vi "Top-V2.2.vi"() -> ()   [LabVIEW 2014]
uses:
  BackMapGlobalV2.2.vi
  ShowMapGlobalV2.2.vi
panel:
  out "Buttom List":string[][](array[string])=[["", "P1", "P2"], ["↑", "\u0000", ""], ["←", "\u0000", ""], ["↓", "", ""], ["→", "", ""], ["☆", "", ""], ["★", "", ""]]
  out "ButtonStringArray":string[](array[string])
  in  "SkipButtonReset?":bool
  out "ButtonArray":i32[](array[numeric])
  out "ButtonSetDone?":bool
  in  "Start":bool
  out "NotFirstClick?":bool
  out "FirstClikPosition":i32[](array[numeric])
  out "Message":string="Please set length, width, number of mines. And press\"SET UP\"."
  in  "Set OK":bool
  out "P2's Score":i32
  out "P1's Score":i32
  out "Mines Remain":i32
  in  "Number of Total Mines":i32(knob)=99 scale=1.0..100.0
  out "SamePlace?":bool
  out "ZeroListBefore":i32[][](array[numeric])
  out "WhichPlayer":i32
  out "ZeroList":i32[][](array[numeric])
  out "BackMap":i32[][](array[numeric])
  in  "Number of Columns":i32(slide)=30 scale=0.0..30.0
  in  "Number of Rows":i32(slide)=16 scale=0.0..16.0
  out "Position":i32[][](array[numeric])=[[0, 1], [1, 0]]
  out "Show Map":cluster{"Color Box":u32, "String":string}[][](array[cluster])=[[{"Color Box"=6908265, "String"=""}]]
  in  "Leave":bool
  out "Char":i16
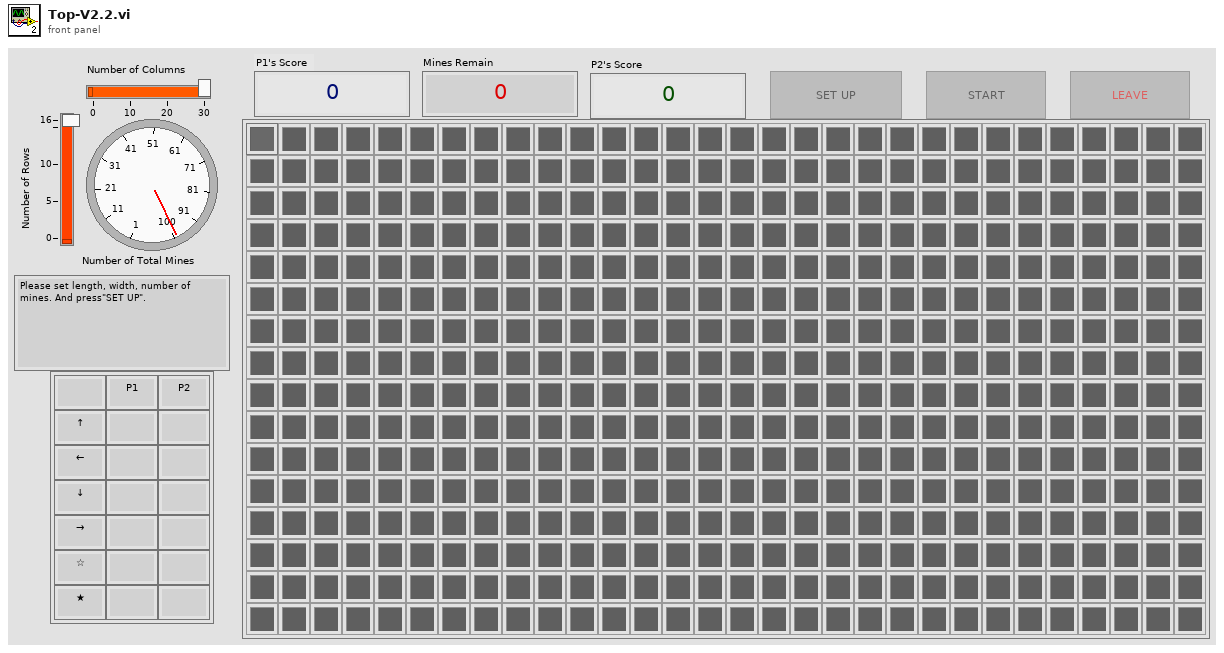
[diagram p1: front panel]
types:
  T1 = enum16{"int", "wait buttom", "w", "a", "s", "d", "q", "e", "i", "j", "k", "l", "u", "o", "spare", "ZeroSpread"}
  T2 = enum8{"Enabled", "Disabled", "Disabled and Grayed Out"}
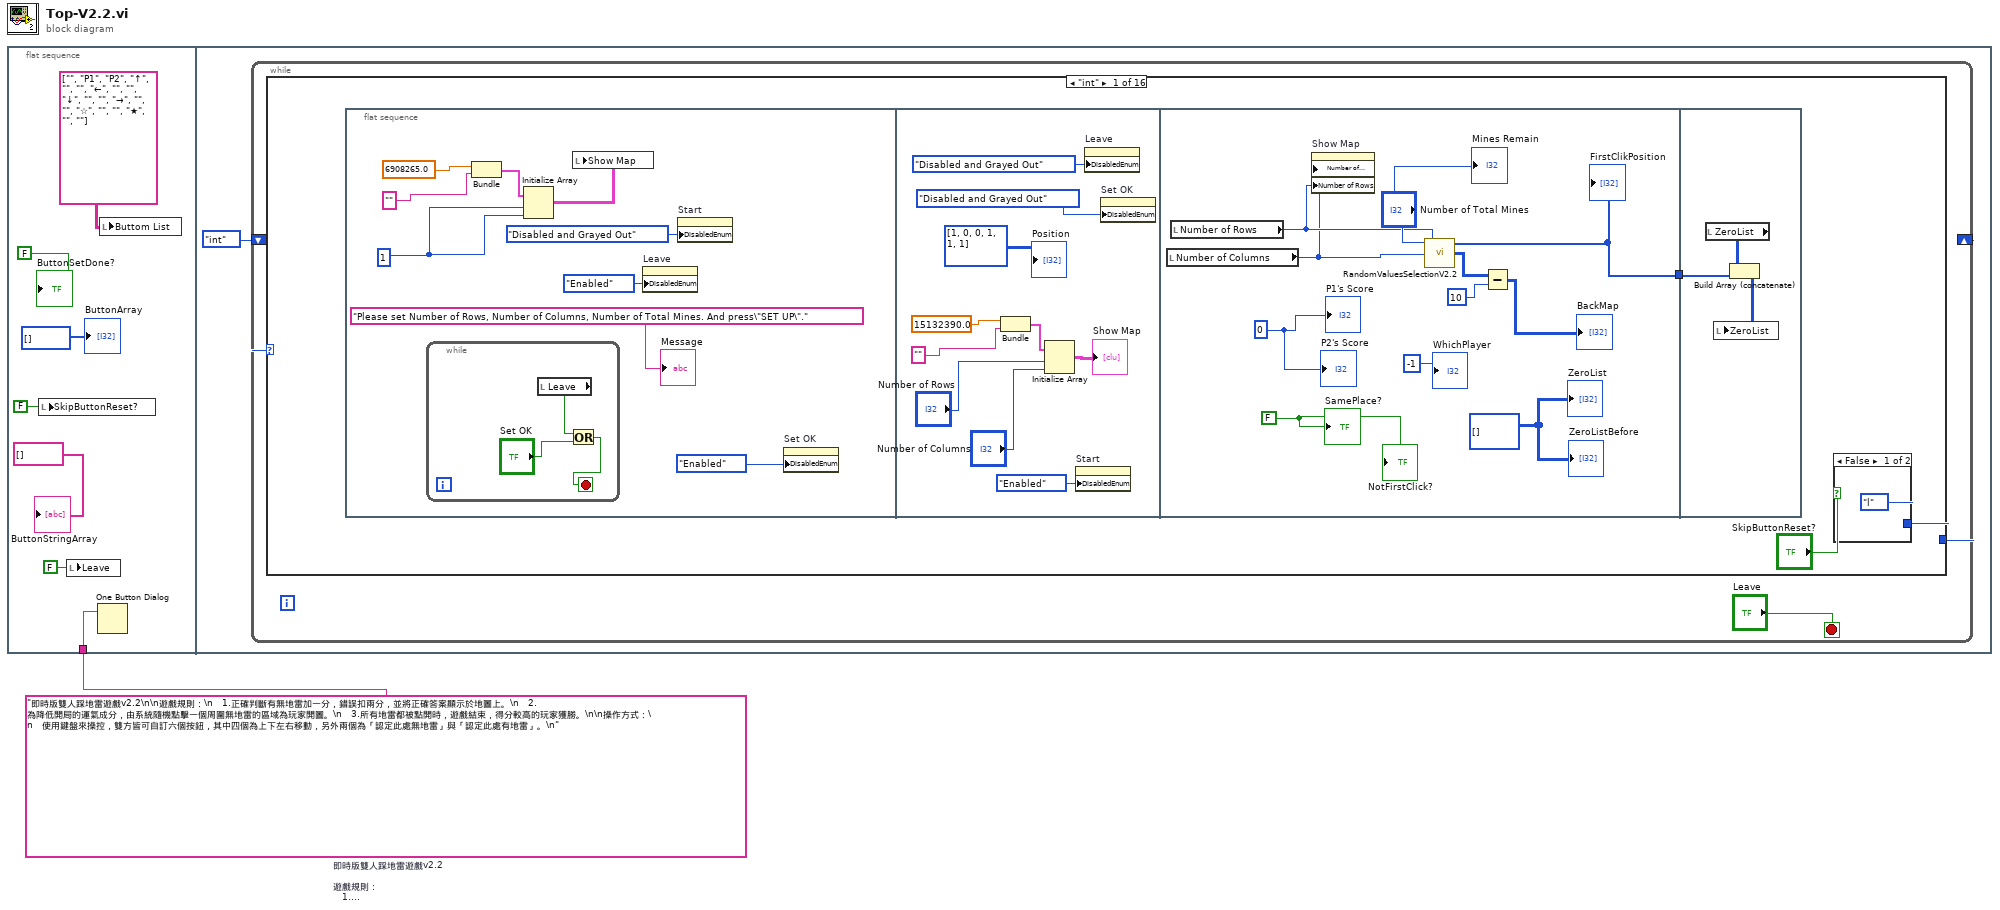
[diagram p0: block diagram]
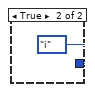
[diagram p2: hidden frame]
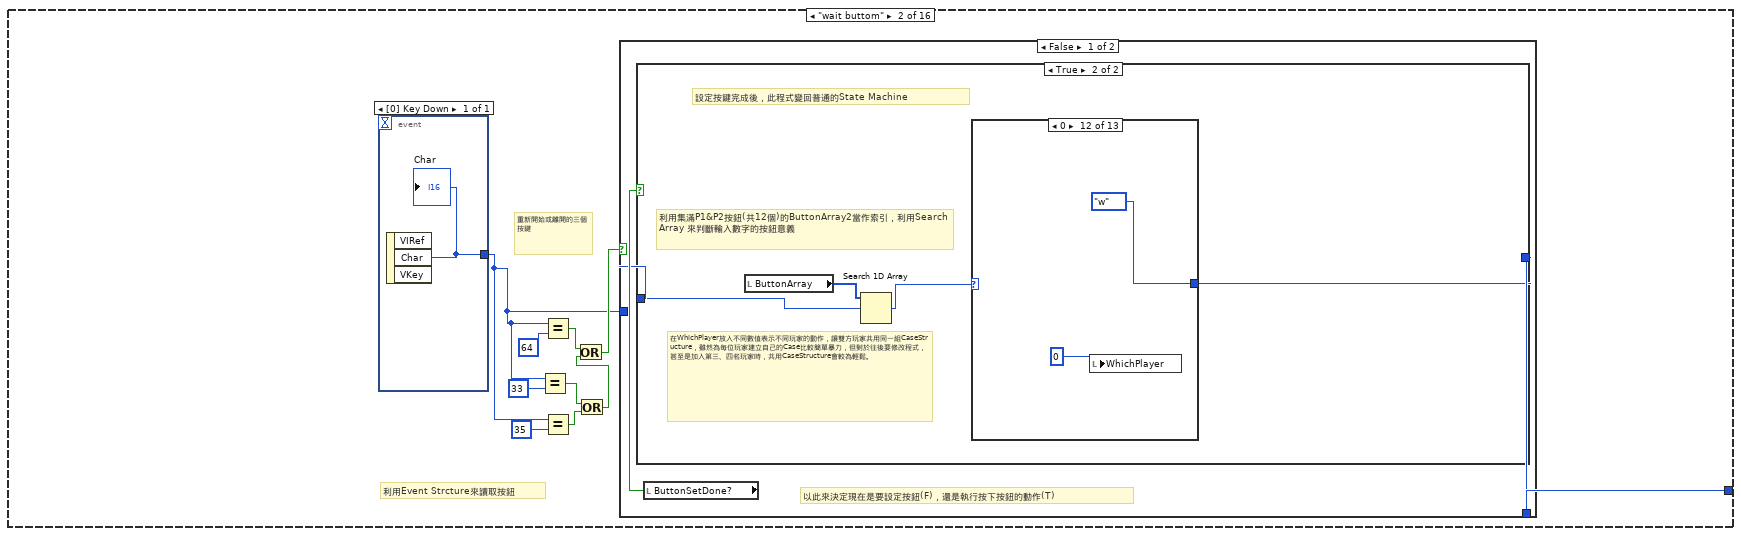
[diagram p3: hidden frame]
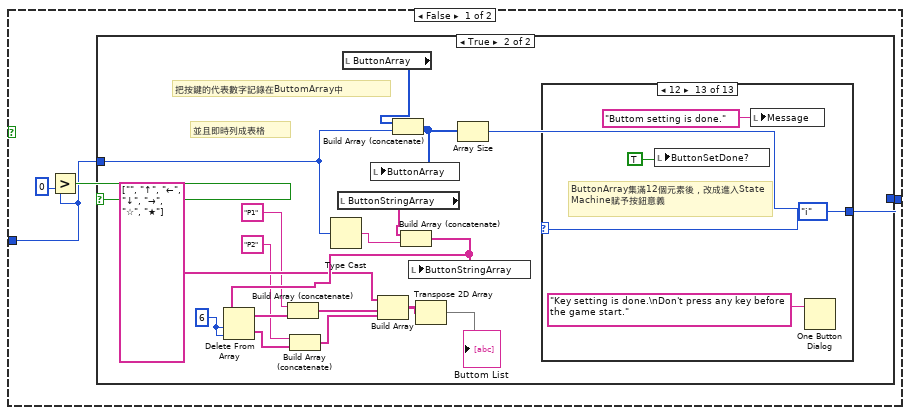
[diagram p4: hidden frame]
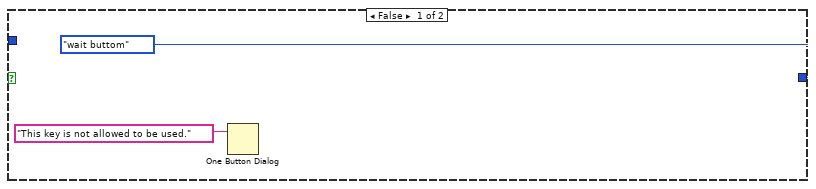
[diagram p5: hidden frame]
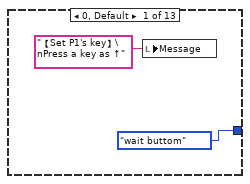
[diagram p6: hidden frame]
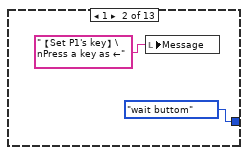
[diagram p7: hidden frame]
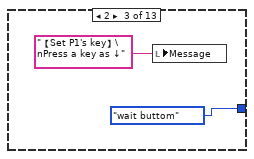
[diagram p8: hidden frame]
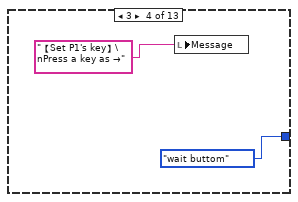
[diagram p9: hidden frame]
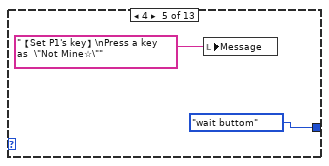
[diagram p10: hidden frame]
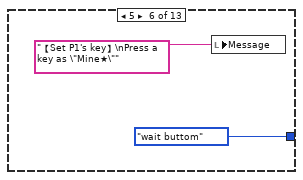
[diagram p11: hidden frame]
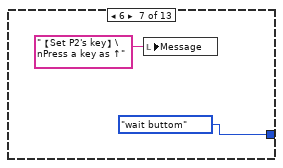
[diagram p12: hidden frame]
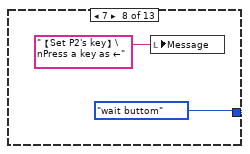
[diagram p13: hidden frame]
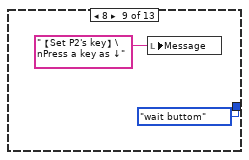
[diagram p14: hidden frame]
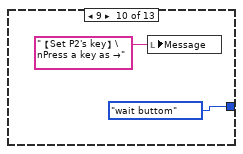
[diagram p15: hidden frame]
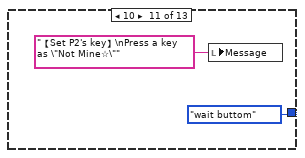
[diagram p16: hidden frame]
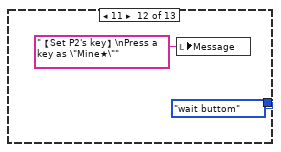
[diagram p17: hidden frame]
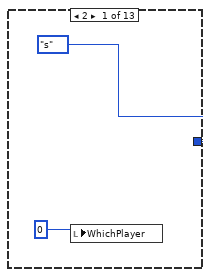
[diagram p18: hidden frame]
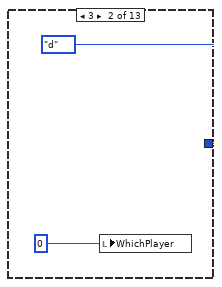
[diagram p19: hidden frame]
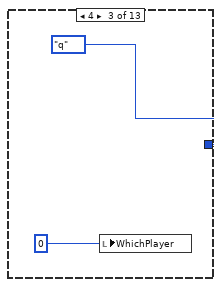
[diagram p20: hidden frame]
diagram:
  w1 = "即時版雙人踩地雷遊戲v2.2\n\n遊戲規則：\n　1.正確判斷有無地雷加一分，錯誤扣兩分，並將正確答案顯示於地圖上。\n　2.為降低開局的運氣成分，由系統隨機點擊一個周圍無地雷的區域為玩家開圖。\n　3.所有地雷都被點開時，遊戲結束，得分較高的玩家獲勝。\n\n操作方式：\n　使用鍵盤來操控，雙方皆可自訂六個按鈕，其中四個為上下左右移動，另外兩個為「認定此處無地雷」與「認定此處有地雷」。\n"  # 即時版雙人踩地雷遊戲v2.2  遊戲規則： 　1.正確判斷有無地雷加一分，錯誤扣兩分，並將正確答案顯示於地圖上。 　2.為降低開局的運氣成分，由系統隨機點擊一個周圍無地雷的區域為玩家開圖。 　3.所有地雷都被點開時，遊戲結束，得分較高的玩家獲勝。  操作方式： 　使用鍵盤來操控，雙方皆可自訂六個按鈕，其中四個為上下左右移動，另外兩個為「認定此處無地雷」與「認定此處有地雷」。
  n1 = flat-sequence {
    tunnel: w1 -> [w4]
    frame #0 {
      n2 = local write "SkipButtonReset?"(FALSE ("SkipButtomReset?")) -> ()
      n3 = local write "Leave"(FALSE ("Leave")) -> ()
      n4 = One Button Dialog(message=w4) -> ()  [unwired: 1 in, 1 out]
      n5 = local write "Buttom List"(string[][] [["", "P1", "P2"], ["↑", "", ""], ["←", "", ""], ["↓", "", ""], ["→", "", ""], ["☆", "", ""], ["★", "", ""]]) -> ()
      "ButtonSetDone?" <- FALSE ("SetButtom?")
      "ButtonArray" <- i32[] []
      "ButtonStringArray" <- string[] []
    }
    frame #1 {
      n6 = while {
        shift-right: [w10] -> _
        shift-left: T1."int" -> [w11]
        stop <- "Leave" stop-if-true
        n7 = case shown="\"int\"" w11 {
          tunnel: [w15 w63 T1."wait buttom" T1."wait buttom" T1."wait buttom" T1."wait buttom" w356 w465 w597 T1."wait buttom" T1."wait buttom" T1."wait buttom" T1."wait buttom" T1."wait buttom" T1."wait buttom" w645] -> w10
          frame "int" {
            n8 = flat-sequence {
              tunnel: [w42] -> w14
              tunnel: w14 -> [w52]
              frame #0 {
                w21 = 1 ("dimension size")
                n9 = while {
                  stop <- w27 stop-if-true
                  n10 = local read "Leave"() -> (w29:bool)
                  n11 = Or(x=w29, y="Set OK") -> (x .or. y?=w27:bool)
                }
                n12 = Bundle(6908265.0, "") -> (w24:cluster{dbl, string})  [unwired: 1 in]
                n13 = Initialize Array(w24, w21, w21) -> (w22:cluster{dbl, string}[][])
                n14 = local write "Show Map"(w22) -> ()
                n15 = property on="Leave" class="Bool (strict)"("DisabledEnum"=T2."Enabled" ("Disabled")) -> ()  [unwired: 2 in, 2 out]
                n16 = property on="Start" class="Bool (strict)"("DisabledEnum"=T2."Disabled and Grayed Out" ("Disabled")) -> ()  [unwired: 2 in, 2 out]
                n17 = property on="Set OK" class="Bool (strict)"("DisabledEnum"=T2."Enabled" ("Disabled")) -> ()  [unwired: 2 in, 2 out]
                "Message" <- "Please set Number of Rows, Number of Columns, Number of Total Mines. And press\"SET UP\"."
              }
              frame #1 {
                n18 = Bundle(15132390.0, "") -> (w37:cluster{dbl, string})  [unwired: 1 in]
                n19 = Initialize Array(w37, "Number of Rows", "Number of Columns") -> (→"Show Map":cluster{dbl, string}[][])
                n20 = property on="Start" class="Bool (strict)"("DisabledEnum"=T2."Enabled" ("Disabled")) -> ()  [unwired: 2 in, 2 out]
                n21 = property on="Leave" class="Bool (strict)"("DisabledEnum"=T2."Disabled and Grayed Out" ("Disabled")) -> ()  [unwired: 2 in, 2 out]
                n22 = property on="Set OK" class="Bool (strict)"("DisabledEnum"=T2."Disabled and Grayed Out" ("Disabled")) -> ()  [unwired: 2 in, 2 out]
                "Position" <- i32[][] [[1, 0], [0, 1], [1, 1]]
              }
              frame #2 {
                w43 = FALSE
                w44 = i32[][] []
                w46 = 0 ("P1's Score")
                n23 = local read "Number of Columns"() -> (w40:i32)
                n24 = local read "Number of Rows"() -> (w41:i32)
                n25 = property on="Show Map" class="Arr (strict)"("Number of Columns"=w40, "Number of Rows"=w41) -> ()  [unwired: 2 in, 2 out]
                n26 = call "RandomValuesSelectionV2.2.vi"("Number of Columns"=w40, "Number of  Rows"=w41, "Number of Mine"="Number of Total Mines") -> ("FullMap"=w48:i32[][], "FirstClikPosition"=w42:i32[])  [unwired: 2 in]
                "FirstClikPosition" <- w42
                n27 = Subtract(x=w48, y=10) -> (x-y=→"BackMap":i32[][])
                "Mines Remain" <- "Number of Total Mines"
                "P1's Score" <- w46
                "P2's Score" <- w46
                "ZeroList" <- w44
                "WhichPlayer" <- -1
                "ZeroListBefore" <- w44
                "SamePlace?" <- w43
                "NotFirstClick?" <- w43
              }
              frame #3 {
                n28 = local read "ZeroList"() -> (w53:i32[][])
                n29 = Build Array (concatenate)(w53, w52) -> (w51:i32[][])
                n30 = local write "ZeroList"(w51) -> ()
              }
            }
            n31 = case shown="False" "SkipButtonReset?" {
              tunnel: [T1."l" T1."i"] -> w15
              frame False {
              }
              frame True {
              }
            }
          }
          frame "wait buttom" {
            # "重新開始或離開的三個按鍵"
            # "利用Event Strcture來讀取按鈕"
            n32 = event shown="[0] Key Down" {
              selector: _ -> [_]
              dyn-events: _ -> [_]
              timeout: _ -> [_]
              tunnel: [w157] -> w58
              event Key Down {
                n33 = event-data() -> ("Char"=w157:i16)  [unwired: 1 in, 2 out]
                "Char" <- w157
              }
            }
            n34 = Equal?(x=w58, y=i16 33) -> (x = y?=w55:bool)
            n35 = Equal?(x=w58, y=i16 64) -> (x = y?=w60:bool)
            n36 = Equal?(x=w58, y=i16 35) -> (x = y?=w56:bool)
            n37 = Or(x=w55, y=w56) -> (x .or. y?=w54:bool)
            n38 = Or(x=w60, y=w54) -> (x .or. y?=w59:bool)
            n39 = case shown="False" w59 {
              tunnel: [w64 w148] -> w63
              tunnel: w58 -> [w65 w149]
              frame False {
                # "以此來決定現在是要設定按鈕(F)，還是執行按下按鈕的動作(T)"
                n40 = local read "ButtonSetDone?"() -> (w66:bool)
                n41 = case shown="True" w66 {
                  tunnel: w65 -> [w68 w120]
                  tunnel: [w67 w122] -> w64
                  frame False {
                    n42 = Greater?(x=w68, y=i16 0) -> (0:w69:bool)
                    n43 = case shown="True" w69 {
                      tunnel: w68 -> [_ w86]
                      tunnel: [T1."wait buttom" w88] -> w67
                      frame False {
                        n44 = One Button Dialog(message="This key is not allowed to be used.") -> ()  [unwired: 1 in, 1 out]
                      }
                      frame True {
                        w82 = 6 ("index")
                        # "並且即時列成表格"
                        # "把按鍵的代表數字記錄在ButtomArray中"
                        n45 = Type Cast(x=w86) -> (*(type *) &x=w84:string)  [unwired: 1 in]
                        n46 = local read "ButtonStringArray"() -> (w85:string[])
                        n47 = local read "ButtonArray"() -> (w90:i32[])
                        n48 = Build Array (concatenate)(w90, w86) -> (w87:i32[])
                        n49 = local write "ButtonArray"(w87) -> ()
                        n50 = Build Array (concatenate)(w85, w84) -> (w83:string[])
                        n51 = Delete From Array(array=w83, length=w82, index=w82) -> (deleted portion=w74:string[], array with subset deleted=w77:string[])
                        n52 = Build Array (concatenate)("P1", w77) -> (w76:string[])
                        n53 = Build Array (concatenate)("P2", w74) -> (w73:string[])
                        n54 = Build Array(string[] ["", "↑", "←", "↓", "→", "☆", "★"], w76, w73) -> (w80:string[][])
                        n55 = local write "ButtonStringArray"(w83) -> ()
                        n56 = Transpose 2D Array(2D array=w80) -> (transposed array=→"Buttom List":string[][])
                        n57 = Array Size(array=w87) -> (size(s)=w89:i32)
                        n58 = case shown="12" w89 {
                          tunnel: [T1."wait buttom" T1."wait buttom" T1."wait buttom" T1."wait buttom" T1."wait buttom" T1."wait buttom" T1."wait buttom" T1."wait buttom" T1."wait buttom" T1."wait buttom" T1."wait buttom" T1."wait buttom" T1."i"] -> w88
                          frame 0, Default {
                            n59 = local write "Message"("【Set P1's key】\nPress a key as ↑" ("Message")) -> ()
                          }
                          frame 1 {
                            n60 = local write "Message"("【Set P1's key】\nPress a key as ←" ("Message")) -> ()
                          }
                          frame 2 {
                            n61 = local write "Message"("【Set P1's key】\nPress a key as ↓" ("Message")) -> ()
                          }
                          frame 3 {
                            n62 = local write "Message"("【Set P1's key】\nPress a key as →" ("Message")) -> ()
                          }
                          frame 4 {
                            n63 = local write "Message"("【Set P1's key】\nPress a key as  \"Not Mine☆\"" ("Message")) -> ()
                          }
                          frame 5 {
                            n64 = local write "Message"("【Set P1's key】\nPress a key as \"Mine★\"" ("Message")) -> ()
                          }
                          frame 6 {
                            n65 = local write "Message"("【Set P2's key】\nPress a key as ↑" ("Message")) -> ()
                          }
                          frame 7 {
                            n66 = local write "Message"("【Set P2's key】\nPress a key as ←" ("Message")) -> ()
                          }
                          frame 8 {
                            n67 = local write "Message"("【Set P2's key】\nPress a key as ↓" ("Message")) -> ()
                          }
                          frame 9 {
                            n68 = local write "Message"("【Set P2's key】\nPress a key as →" ("Message")) -> ()
                          }
                          frame 10 {
                            n69 = local write "Message"("【Set P2's key】\nPress a key as \"Not Mine☆\"" ("Message")) -> ()
                          }
                          frame 11 {
                            n70 = local write "Message"("【Set P2's key】\nPress a key as \"Mine★\"" ("Message")) -> ()
                          }
                          frame 12 {
                            # "ButtonArray集滿12個元素後，改成進入State Machine賦予按鈕意義"
                            n71 = local write "ButtonSetDone?"(TRUE ("SetButtom?")) -> ()
                            n72 = local write "Message"("Buttom setting is done." ("Message")) -> ()
                            n73 = One Button Dialog(message="Key setting is done.\nDon't press any key before the game start.") -> ()  [unwired: 1 in, 1 out]
                          }
                        }
                      }
                    }
                  }
                  frame True {
                    # "在WhichPlayer放入不同數值表示不同玩家的動作，讓雙方玩家共用同一組CaseStructure，雖然為每位玩家建立自己的Case比較簡單暴力，但對於往後要修改程式，甚至是加入第三、四名玩家時，共用CaseStructure會較為輕鬆。"
                    # "利用集滿P1&P2按鈕(共12個)的ButtonArray2當作索引，利用Search Array 來判斷輸入數字的按鈕意義"
                    # "設定按鍵完成後，此程式變回普通的State Machine"
                    n74 = local read "ButtonArray"() -> (w121:i32[])
                    n75 = Search 1D Array(1D array=w121, element=w120) -> (index of element=w119:i32)  [unwired: 1 in]
                    n76 = case shown="0" w119 {
                      tunnel: [T1."s" T1."d" T1."q" T1."e" T1."w" T1."a" T1."s" T1."d" T1."q" T1."e" T1."wait buttom" T1."w" T1."a"] -> w122
                      frame 2 {
                        n77 = local write "WhichPlayer"(0 ("WhichPlayer")) -> ()
                      }
                      frame 3 {
                        n78 = local write "WhichPlayer"(0 ("WhichPlayer")) -> ()
                      }
                      frame 4 {
                        n79 = local write "WhichPlayer"(0 ("WhichPlayer")) -> ()
                      }
                      frame 5 {
                        n80 = local write "WhichPlayer"(0 ("WhichPlayer")) -> ()
                      }
                      frame 6 {
                        n81 = local write "WhichPlayer"(1 ("WhichPlayer")) -> ()
                      }
                      frame 7 {
                        n82 = local write "WhichPlayer"(1 ("WhichPlayer")) -> ()
                      }
                      frame 8 {
                        n83 = local write "WhichPlayer"(1 ("WhichPlayer")) -> ()
                      }
                      frame 9 {
                        n84 = local write "WhichPlayer"(1 ("WhichPlayer")) -> ()
                      }
                      frame 10 {
                        n85 = local write "WhichPlayer"(1 ("WhichPlayer")) -> ()
                      }
                      frame 11 {
                        n86 = local write "WhichPlayer"(1 ("WhichPlayer")) -> ()
                      }
                      frame -1, Default {
                      }
                      frame 0 {
                        n87 = local write "WhichPlayer"(0 ("WhichPlayer")) -> ()
                      }
                      frame 1 {
                        n88 = local write "WhichPlayer"(0 ("WhichPlayer")) -> ()
                      }
                    }
                  }
                }
              }
              frame True {
                n89 = case shown="35" w149 {
                  tunnel: [T1."spare" T1."int" T1."wait buttom" T1."int"] -> w148
                  frame 64 {
                    n90 = local write "Leave"(TRUE ("Leave")) -> ()
                  }
                  frame 35 {
                    n91 = local write "SkipButtonReset?"(TRUE ("SkipButtomReset?")) -> ()
                  }
                  frame -1, Default {
                  }
                  frame 33 {
                    n92 = local write "SkipButtonReset?"(FALSE ("SkipButtomReset?")) -> ()
                  }
                }
              }
            }
          }
          frame "w" {
            n93 = flat-sequence {
              tunnel: [w170] -> w159
              tunnel: w159 -> [w193]
              tunnel: [w193] -> w158
              tunnel: w158 -> [w197]
              frame #0 {
                n94 = local read "WhichPlayer"() -> (w161:i32)
                n95 = local read "BackMap"() -> (w164:i32[][])
                n96 = local read "Position"() -> (w171:i32[][])
                n97 = local read "SamePlace?"() -> (w168:bool)
                n98 = Index Array(array=w171, index (row) #1=w161, index (col) #1=0 ("index (row)"), index (row) #2=w161, index (col) #2=1 ("disabled index (col)")) -> (element #1=w163:i32, element #2=w162:i32)
                n99 = call "AfterSamePositionColor-V2.2.vi"("WhichPlayer"=w161, "index (col)"=w162, "index (row)"=w163, "BackMap"=w164) -> ("Numeric"=w167:dbl)  [unwired: 2 in]
                n100 = call "ToBackMap-V2.2.vi"("Column"=w162, "Row"=w163, "BackMap"=w164) -> ("String"=w169:string, "Numeric"=w166:dbl)  [unwired: 2 in]
                n101 = Select(t=w167, s=w168, f=w166) -> (s? t:f=w165:dbl)
                n102 = Greater?(x=w163, y=0) -> (0:w174:bool)
                n103 = case shown="True" w174 {
                  tunnel: w163 -> [_ w191]
                  tunnel: w171 -> [w176 w182]
                  tunnel: [w176 w188] -> w170
                  tunnel: w165 -> [_ w179]
                  tunnel: w169 -> [_ w178]
                  tunnel: w161 -> [_ w177]
                  frame False {
                  }
                  frame True {
                    n104 = Decrement(x=w191) -> (x-1=w189:i32)
                    n105 = local read "Show Map"() -> (w181:cluster{"Color Box":u32, "String":string}[][])
                    n106 = Bundle("Numeric"=w179, "String"=w178) -> (w183:cluster{"Numeric":dbl, "String":string})  [unwired: 1 in]
                    n107 = Index Array(array=w182, index (row) #1=w177, index (col) #1=0 ("index (row)"), index (row) #2=w177, index (col) #2=1 ("disabled index (col)")) -> (element #1=w186:i32, element #2=w187:i32)
                    n108 = Replace Array Subset(array=w182, new element=w189, index (row)=w177, index (col)=0 ("index (row)")) -> (w188:i32[][])
                    n109 = Replace Array Subset(array=w181, new element=w183, index (row)=w186, index (col)=w187) -> (w180:cluster{"Color Box":u32, "String":string}[][])
                    n110 = local write "Show Map"(w180) -> ()
                  }
                }
              }
              frame #1 {
                n111 = local write "SamePlace?"(FALSE ("SamePlace?")) -> ()
              }
              frame #2 {
                n112 = local read "WhichPlayer"() -> (w198:i32)
                n113 = local write "Position"(w197) -> ()
                n114 = local read "BackMap"() -> (w202:i32[][])
                n115 = Index Array(array=w197, index (row) #1=w198, index (col) #1=0 ("index (row)"), index (row) #2=w198, index (col) #2=1 ("disabled index (col)")) -> (element #1=w201:i32, element #2=w200:i32)
                n116 = call "ZeroOrNot-V2.2.vi"("WhichPlayer"=w198, "index (col)"=w200, "index (row)"=w201, "BackMap"=w202) -> ("Numeric"=w196:dbl)  [unwired: 2 in]
                n117 = call "PositionSameOrNot-V2.2.vi"("BlueOrGreen"=w196, "Position"=w197) -> ("SamePosition?"=w194:bool, "FinalColor"=w195:dbl)  [unwired: 1 in]
                n118 = local read "Show Map"() -> (w206:cluster{"Color Box":u32, "String":string}[][])
                n119 = local write "SamePlace?"(w194) -> ()
                n120 = call "ToBackMap-V2.2.vi"("Column"=w200, "Row"=w201, "BackMap"=w202) -> ("String"=w203:string)  [unwired: 2 in, 1 out]
                n121 = Bundle("FinalColor"=w195, "String"=w203) -> (w205:cluster{"FinalColor":dbl, "String":string})  [unwired: 1 in]
                n122 = Replace Array Subset(array=w206, new element=w205, index (row)=w201, index (col)=w200) -> (w207:cluster{"Color Box":u32, "String":string}[][])
                n123 = local write "Show Map"(w207) -> ()
              }
            }
          }
          frame "a" {
            n124 = flat-sequence {
              tunnel: [w221] -> w209
              tunnel: w209 -> [w241]
              tunnel: [w241] -> w208
              tunnel: w208 -> [w245]
              frame #0 {
                n125 = local read "BackMap"() -> (w216:i32[][])
                n126 = local read "WhichPlayer"() -> (w213:i32)
                n127 = local read "SamePlace?"() -> (w218:bool)
                n128 = local read "Position"() -> (w222:i32[][])
                n129 = Index Array(array=w222, index (row) #1=w213, index (col) #1=0 ("index (row)"), index (row) #2=w213, index (col) #2=1 ("disabled index (col)")) -> (element #1=w214:i32, element #2=w215:i32)
                n130 = call "AfterSamePositionColor-V2.2.vi"("WhichPlayer"=w213, "index (col)"=w215, "index (row)"=w214, "BackMap"=w216) -> ("Numeric"=w217:dbl)  [unwired: 2 in]
                n131 = call "ToBackMap-V2.2.vi"("Column"=w215, "Row"=w214, "BackMap"=w216) -> ("String"=w219:string, "Numeric"=w212:dbl)  [unwired: 2 in]
                n132 = Select(t=w217, s=w218, f=w212) -> (s? t:f=w211:dbl)
                n133 = Greater?(x=w215, y=0) -> (0:w225:bool)
                n134 = case shown="True" w225 {
                  tunnel: w215 -> [_ w239]
                  tunnel: w222 -> [w226 w236]
                  tunnel: [w226 w237] -> w221
                  tunnel: w214 -> [_ w235]
                  tunnel: w215 -> [_ w234]
                  tunnel: w211 -> [_ w229]
                  tunnel: w219 -> [_ w228]
                  tunnel: w213 -> [_ w227]
                  frame False {
                  }
                  frame True {
                    n135 = local read "Show Map"() -> (w233:cluster{"Color Box":u32, "String":string}[][])
                    n136 = Decrement(x=w239) -> (x-1=w238:i32)
                    n137 = Bundle("Numeric"=w229, "String"=w228) -> (w232:cluster{"Numeric":dbl, "String":string})  [unwired: 1 in]
                    n138 = Replace Array Subset(array=w236, new element=w238, index (row)=w227, index (col)=1 ("disabled index (col)")) -> (w237:i32[][])
                    n139 = Replace Array Subset(array=w233, new element=w232, index (row)=w235, index (col)=w234) -> (w231:cluster{"Color Box":u32, "String":string}[][])
                    n140 = local write "Show Map"(w231) -> ()
                  }
                }
              }
              frame #1 {
                n141 = local write "SamePlace?"(FALSE ("SamePlace?")) -> ()
              }
              frame #2 {
                n142 = local read "WhichPlayer"() -> (w246:i32)
                n143 = local read "BackMap"() -> (w249:i32[][])
                n144 = local write "Position"(w245) -> ()
                n145 = Index Array(array=w245, index (row) #1=w246, index (col) #1=0 ("index (row)"), index (row) #2=w246, index (col) #2=1 ("disabled index (col)")) -> (element #1=w248:i32, element #2=w247:i32)
                n146 = call "ZeroOrNot-V2.2.vi"("WhichPlayer"=w246, "index (col)"=w247, "index (row)"=w248, "BackMap"=w249) -> ("Numeric"=w244:dbl)  [unwired: 2 in]
                n147 = call "PositionSameOrNot-V2.2.vi"("BlueOrGreen"=w244, "Position"=w245) -> ("SamePosition?"=w242:bool, "FinalColor"=w243:dbl)  [unwired: 1 in]
                n148 = local read "Show Map"() -> (w254:cluster{"Color Box":u32, "String":string}[][])
                n149 = call "ToBackMap-V2.2.vi"("Column"=w247, "Row"=w248, "BackMap"=w249) -> ("String"=w250:string)  [unwired: 2 in, 1 out]
                n150 = local write "SamePlace?"(w242) -> ()
                n151 = Bundle("FinalColor"=w243, "String"=w250) -> (w253:cluster{"FinalColor":dbl, "String":string})  [unwired: 1 in]
                n152 = Replace Array Subset(array=w254, new element=w253, index (row)=w248, index (col)=w247) -> (w255:cluster{"Color Box":u32, "String":string}[][])
                n153 = local write "Show Map"(w255) -> ()
              }
            }
          }
          frame "s" {
            n154 = flat-sequence {
              tunnel: [w270] -> w257
              tunnel: w257 -> [w290]
              tunnel: [w290] -> w256
              tunnel: w256 -> [w294]
              frame #0 {
                n155 = local read "WhichPlayer"() -> (w259:i32)
                n156 = local read "BackMap"() -> (w262:i32[][])
                n157 = local read "SamePlace?"() -> (w266:bool)
                n158 = local read "Position"() -> (w271:i32[][])
                n159 = local read "Number of Rows"() -> (w269:i32)
                n160 = Index Array(array=w271, index (row) #1=w259, index (col) #1=0 ("index (row)"), index (row) #2=w259, index (col) #2=1 ("disabled index (col)")) -> (element #1=w261:i32, element #2=w260:i32)
                n161 = call "AfterSamePositionColor-V2.2.vi"("WhichPlayer"=w259, "index (col)"=w260, "index (row)"=w261, "BackMap"=w262) -> ("Numeric"=w265:dbl)  [unwired: 2 in]
                n162 = call "ToBackMap-V2.2.vi"("Column"=w260, "Row"=w261, "BackMap"=w262) -> ("String"=w267:string, "Numeric"=w264:dbl)  [unwired: 2 in]
                n163 = Select(t=w265, s=w266, f=w264) -> (s? t:f=w263:dbl)
                n164 = Decrement(x=w269) -> (x-1=w268:i32)
                n165 = Less?(x=w261, y=w268) -> (x < y?=w274:bool)
                n166 = case shown="True" w274 {
                  tunnel: w261 -> [_ w288]
                  tunnel: w271 -> [w275 w284]
                  tunnel: [w275 w285] -> w270
                  tunnel: w261 -> [_ w283]
                  tunnel: w260 -> [_ w282]
                  tunnel: w263 -> [_ w278]
                  tunnel: w267 -> [_ w277]
                  tunnel: w259 -> [_ w276]
                  frame False {
                  }
                  frame True {
                    n167 = Increment(x=w288) -> (x+1=w286:i32)
                    n168 = local read "Show Map"() -> (w281:cluster{"Color Box":u32, "String":string}[][])
                    n169 = Bundle("Numeric"=w278, "String"=w277) -> (w280:cluster{"Numeric":dbl, "String":string})  [unwired: 1 in]
                    n170 = Replace Array Subset(array=w284, new element=w286, index (row)=w276, index (col)=0 ("index (row)")) -> (w285:i32[][])
                    n171 = Replace Array Subset(array=w281, new element=w280, index (row)=w283, index (col)=w282) -> (w279:cluster{"Color Box":u32, "String":string}[][])
                    n172 = local write "Show Map"(w279) -> ()
                  }
                }
              }
              frame #1 {
                n173 = local write "SamePlace?"(FALSE ("SamePlace?")) -> ()
              }
              frame #2 {
                n174 = local read "WhichPlayer"() -> (w295:i32)
                n175 = local write "Position"(w294) -> ()
                n176 = Index Array(array=w294, index (row) #1=w295, index (col) #1=0 ("index (row)"), index (row) #2=w295, index (col) #2=1 ("disabled index (col)")) -> (element #1=w297:i32, element #2=w296:i32)
                n177 = local read "BackMap"() -> (w298:i32[][])
                n178 = local read "Show Map"() -> (w303:cluster{"Color Box":u32, "String":string}[][])
                n179 = call "ZeroOrNot-V2.2.vi"("WhichPlayer"=w295, "index (col)"=w296, "index (row)"=w297, "BackMap"=w298) -> ("Numeric"=w293:dbl)  [unwired: 2 in]
                n180 = call "PositionSameOrNot-V2.2.vi"("BlueOrGreen"=w293, "Position"=w294) -> ("SamePosition?"=w291:bool, "FinalColor"=w292:dbl)  [unwired: 1 in]
                n181 = local write "SamePlace?"(w291) -> ()
                n182 = call "ToBackMap-V2.2.vi"("Column"=w296, "Row"=w297, "BackMap"=w298) -> ("String"=w299:string)  [unwired: 2 in, 1 out]
                n183 = Bundle("FinalColor"=w292, "String"=w299) -> (w302:cluster{"FinalColor":dbl, "String":string})  [unwired: 1 in]
                n184 = Replace Array Subset(array=w303, new element=w302, index (row)=w297, index (col)=w296) -> (w304:cluster{"Color Box":u32, "String":string}[][])
                n185 = local write "Show Map"(w304) -> ()
              }
            }
          }
          frame "d" {
            n186 = flat-sequence {
              tunnel: [w319] -> w306
              tunnel: w306 -> [w339]
              tunnel: [w339] -> w305
              tunnel: w305 -> [w343]
              frame #0 {
                n187 = local read "BackMap"() -> (w311:i32[][])
                n188 = local read "WhichPlayer"() -> (w310:i32)
                n189 = local read "SamePlace?"() -> (w315:bool)
                n190 = local read "Number of Columns"() -> (w318:i32)
                n191 = local read "Position"() -> (w320:i32[][])
                n192 = Index Array(array=w320, index (row) #1=w310, index (col) #1=0 ("index (row)"), index (row) #2=w310, index (col) #2=1 ("disabled index (col)")) -> (element #1=w309:i32, element #2=w308:i32)
                n193 = call "AfterSamePositionColor-V2.2.vi"("WhichPlayer"=w310, "index (col)"=w308, "index (row)"=w309, "BackMap"=w311) -> ("Numeric"=w314:dbl)  [unwired: 2 in]
                n194 = Decrement(x=w318) -> (x-1=w317:i32)
                n195 = call "ToBackMap-V2.2.vi"("Column"=w308, "Row"=w309, "BackMap"=w311) -> ("String"=w316:string, "Numeric"=w313:dbl)  [unwired: 2 in]
                n196 = Select(t=w314, s=w315, f=w313) -> (s? t:f=w312:dbl)
                n197 = Less?(x=w308, y=w317) -> (x < y?=w323:bool)
                n198 = case shown="True" w323 {
                  tunnel: w308 -> [_ w337]
                  tunnel: w320 -> [w324 w334]
                  tunnel: [w324 w335] -> w319
                  tunnel: w309 -> [_ w333]
                  tunnel: w308 -> [_ w332]
                  tunnel: w312 -> [_ w327]
                  tunnel: w316 -> [_ w326]
                  tunnel: w310 -> [_ w325]
                  frame False {
                  }
                  frame True {
                    n199 = Increment(x=w337) -> (x+1=w336:i32)
                    n200 = local read "Show Map"() -> (w331:cluster{"Color Box":u32, "String":string}[][])
                    n201 = Bundle("Numeric"=w327, "String"=w326) -> (w330:cluster{"Numeric":dbl, "String":string})  [unwired: 1 in]
                    n202 = Replace Array Subset(array=w334, new element=w336, index (row)=w325, index (col)=1 ("disabled index (col)")) -> (w335:i32[][])
                    n203 = Replace Array Subset(array=w331, new element=w330, index (row)=w333, index (col)=w332) -> (w329:cluster{"Color Box":u32, "String":string}[][])
                    n204 = local write "Show Map"(w329) -> ()
                  }
                }
              }
              frame #1 {
                n205 = local write "SamePlace?"(FALSE ("SamePlace?")) -> ()
              }
              frame #2 {
                n206 = local read "WhichPlayer"() -> (w344:i32)
                n207 = local read "BackMap"() -> (w347:i32[][])
                n208 = Index Array(array=w343, index (row) #1=w344, index (col) #1=0 ("index (row)"), index (row) #2=w344, index (col) #2=1 ("disabled index (col)")) -> (element #1=w346:i32, element #2=w345:i32)
                n209 = call "ZeroOrNot-V2.2.vi"("WhichPlayer"=w344, "index (col)"=w345, "index (row)"=w346, "BackMap"=w347) -> ("Numeric"=w342:dbl)  [unwired: 2 in]
                n210 = call "PositionSameOrNot-V2.2.vi"("BlueOrGreen"=w342, "Position"=w343) -> ("SamePosition?"=w340:bool, "FinalColor"=w341:dbl)  [unwired: 1 in]
                n211 = local write "SamePlace?"(w340) -> ()
                n212 = local read "BackMap"() -> (w349:i32[][])
                n213 = local read "Show Map"() -> (w353:cluster{"Color Box":u32, "String":string}[][])
                n214 = call "ToBackMap-V2.2.vi"("Column"=w345, "Row"=w346, "BackMap"=w349) -> ("String"=w348:string)  [unwired: 2 in, 1 out]
                n215 = Bundle("FinalColor"=w341, "String"=w348) -> (w352:cluster{"FinalColor":dbl, "String":string})  [unwired: 1 in]
                n216 = local write "Position"(w343) -> ()
                n217 = Replace Array Subset(array=w353, new element=w352, index (row)=w346, index (col)=w345) -> (w354:cluster{"Color Box":u32, "String":string}[][])
                n218 = local write "Show Map"(w354) -> ()
              }
            }
          }
          frame "q" {
            n219 = local read "WhichPlayer"() -> (w355:i32)
            n220 = local read "Position"() -> (w365:i32[][])
            n221 = local read "BackMap"() -> (w362:i32[][])
            n222 = Index Array(array=w365, index (row) #1=w355, index (col) #1=0 ("index (row)"), index (row) #2=w355, index (col) #2=1 ("disabled index (col)")) -> (element #1=w358:i32, element #2=w357:i32)
            n223 = Index Array(array=w362, index (row)=w358, index (col)=w357) -> (element=w359:i32)
            n224 = Less?(x=w359, y=0) -> (x < y?=w360:bool)
            n225 = case shown="True" w360 {
              tunnel: w359 -> [_ w375]
              tunnel: w358 -> [_ w369]
              tunnel: w357 -> [_ w370]
              tunnel: [T1."wait buttom" w367] -> w356
              frame False {
              }
              frame True {
                n226 = local read "BackMap"() -> (w376:i32[][])
                n227 = Add(x=w375, y=10) -> (x+y=w368:i32)
                n228 = Replace Array Subset(array=w376, new element=w368, index (row)=w369, index (col)=w370) -> (w373:i32[][])
                n229 = local write "BackMap"(w373) -> ()
                n230 = Equal?(x=w368, y=9) -> (x = y?=w371:bool)
                n231 = case shown="False" w371 {
                  tunnel: w370 -> [w382 w426]
                  tunnel: w369 -> [w383 w425]
                  tunnel: w368 -> [w381 _]
                  tunnel: [w380 w420] -> w367
                  frame False {
                    n232 = local read "WhichPlayer"() -> (w379:i32)
                    n233 = case shown="1" w379 {
                      tunnel: [460139.0 1199628.0] -> w378
                      tunnel: [5866239.0 6678103.0] -> w377
                      frame 0, Default {
                        n234 = local read "P1's Score"() -> (w389:i32)
                        n235 = Increment(x=w389) -> (x+1=w388:i32)
                        n236 = local write "P1's Score"(w388) -> ()
                      }
                      frame 1 {
                        n237 = local read "P2's Score"() -> (w393:i32)
                        n238 = Increment(x=w393) -> (x+1=w392:i32)
                        n239 = local write "P2's Score"(w392) -> ()
                      }
                    }
                    n240 = Equal?(x=w381, y=0) -> (x = y?=w384:bool)
                    n241 = case shown="True" w384 {
                      tunnel: w383 -> [w398 w416]
                      tunnel: w382 -> [w397 w415]
                      tunnel: w381 -> [w402 _]
                      tunnel: [T1."wait buttom" T1."ZeroSpread"] -> w380
                      tunnel: w379 -> [_ w404]
                      tunnel: w378 -> [_ w403]
                      tunnel: w377 -> [w394 _]
                      frame False {
                        n242 = Number To Decimal String(number=w402) -> (decimal integer string=w400:string)  [unwired: 1 in]
                        n243 = local read "Show Map"() -> (w399:cluster{"Color Box":u32, "String":string}[][])
                        n244 = Bundle(w394, w400) -> (w401:cluster{dbl, string})  [unwired: 1 in]
                        n245 = Replace Array Subset(array=w399, new element=w401, index (row)=w398, index (col)=w397) -> (w396:cluster{"Color Box":u32, "String":string}[][])
                        n246 = local write "Show Map"(w396) -> ()
                      }
                      frame True {
                        n247 = local read "Show Map"() -> (w414:cluster{"Color Box":u32, "String":string}[][])
                        n248 = Bundle(w403, "") -> (w417:cluster{dbl, string})  [unwired: 1 in]
                        n249 = Replace Array Subset(array=w414, new element=w417, index (row)=w416, index (col)=w415) -> (w413:cluster{"Color Box":u32, "String":string}[][])
                        n250 = local write "Show Map"(w413) -> ()
                        n251 = local read "Position"() -> (w411:i32[][])
                        n252 = local read "ZeroList"() -> (w406:i32[][])
                        n253 = Array Subset(array=w411, index (row)=w404, length (row)=1 ("length"), index (col)=0 ("index"), length (col)=2 ("length")) -> (w407:i32[][])
                        n254 = Build Array (concatenate)(w407, w406) -> (w405:i32[][])
                        n255 = local write "ZeroList"(w405) -> ()
                      }
                    }
                  }
                  frame True {
                    n256 = flat-sequence {
                      tunnel: w426 -> [w432]
                      tunnel: w425 -> [w433]
                      tunnel: [w433] -> w424
                      tunnel: [w432] -> w422
                      tunnel: w424 -> [w449]
                      tunnel: [w449] -> w423
                      tunnel: w422 -> [w448]
                      tunnel: [w448] -> w421
                      tunnel: w423 -> [w457]
                      tunnel: w421 -> [w456]
                      tunnel: [w451] -> w419
                      frame #0 {
                        n257 = local read "Mines Remain"() -> (w431:i32)
                        n258 = Decrement(x=w431) -> (x-1=w430:i32)
                        n259 = local write "Mines Remain"(w430) -> ()
                        n260 = local read "WhichPlayer"() -> (w429:i32)
                        n261 = local read "Show Map"() -> (w437:cluster{"Color Box":u32, "String":string}[][])
                        n262 = case shown="0, Default" w429 {
                          frame 0, Default {
                            n263 = local read "P1's Score"() -> (w442:i32)
                            n264 = Subtract(x=w442, y=2) -> (x-y=w441:i32)
                            n265 = local write "P1's Score"(w441) -> ()
                            n266 = property on="P1's Score" class="DigNum (strict)"("NumText.BGColor"=u32 16711680 ("Label.Colors:BG Color")) -> ()  [unwired: 2 in, 2 out]
                          }
                          frame 1 {
                            n267 = local read "P2's Score"() -> (w446:i32)
                            n268 = Subtract(x=w446, y=2) -> (x-y=w445:i32)
                            n269 = local write "P2's Score"(w445) -> ()
                            n270 = property on="P2's Score" class="DigNum (strict)"("NumText.BGColor"=u32 16711680 ("Numeric Text.Text Colors:BG Color")) -> ()  [unwired: 2 in, 2 out]
                          }
                        }
                        n271 = Bundle(16711680.0, "★") -> (w434:cluster{dbl, string})  [unwired: 1 in]
                        n272 = Replace Array Subset(array=w437, new element=w434, index (row)=w433, index (col)=w432) -> (w438:cluster{"Color Box":u32, "String":string}[][])
                        n273 = local write "Show Map"(w438) -> ()
                      }
                      frame #1 {
                        n274 = Wait Until Next ms Multiple(millisecond multiple=u32 1000) -> ()  [unwired: 1 out]
                      }
                      frame #2 {
                        w450 = u32 15132390 ("Label.Colors:BG Color")
                        n275 = local read "WhichPlayer"() -> (w454:i32)
                        n276 = case shown="1" w454 {
                          tunnel: [5866239.0 6678103.0] -> w460
                          frame 0, Default {
                          }
                          frame 1 {
                          }
                        }
                        n277 = property on="P1's Score" class="DigNum (strict)"("NumText.BGColor"=w450) -> ()  [unwired: 2 in, 2 out]
                        n278 = local read "Show Map"() -> (w458:cluster{"Color Box":u32, "String":string}[][])
                        n279 = local read "Mines Remain"() -> (w453:i32)
                        n280 = Bundle(w460, "★") -> (w459:cluster{dbl, string})  [unwired: 1 in]
                        n281 = property on="P2's Score" class="DigNum (strict)"("NumText.BGColor"=w450) -> ()  [unwired: 2 in, 2 out]
                        n282 = Replace Array Subset(array=w458, new element=w459, index (row)=w457, index (col)=w456) -> (w455:cluster{"Color Box":u32, "String":string}[][])
                        n283 = local write "Show Map"(w455) -> ()
                        n284 = Equal?(x=w453, y=0) -> (x = y?=w451:bool)
                      }
                    }
                    n285 = case shown="False" w419 {
                      tunnel: [T1."wait buttom" T1."k"] -> w420
                      frame False {
                      }
                      frame True {
                      }
                    }
                  }
                }
              }
            }
          }
          frame "e" {
            n286 = local read "WhichPlayer"() -> (w464:i32)
            n287 = local read "Position"() -> (w474:i32[][])
            n288 = local read "BackMap"() -> (w471:i32[][])
            n289 = Index Array(array=w474, index (row) #1=w464, index (col) #1=0 ("index (row)"), index (row) #2=w464, index (col) #2=1 ("disabled index (col)")) -> (element #1=w467:i32, element #2=w466:i32)
            n290 = Index Array(array=w471, index (row)=w467, index (col)=w466) -> (element=w468:i32)
            n291 = Less?(x=w468, y=0) -> (x < y?=w469:bool)
            n292 = case shown="True" w469 {
              tunnel: w468 -> [_ w484]
              tunnel: w467 -> [_ w478]
              tunnel: w466 -> [_ w479]
              tunnel: [T1."wait buttom" w476] -> w465
              frame False {
              }
              frame True {
                n293 = local read "BackMap"() -> (w485:i32[][])
                n294 = Add(x=w484, y=10) -> (x+y=w477:i32)
                n295 = Replace Array Subset(array=w485, new element=w477, index (row)=w478, index (col)=w479) -> (w482:i32[][])
                n296 = local write "BackMap"(w482) -> ()
                n297 = Equal?(x=w477, y=9) -> (x = y?=w480:bool)
                n298 = case shown="False" w480 {
                  tunnel: w479 -> [w491 w582]
                  tunnel: w478 -> [w492 w583]
                  tunnel: w477 -> [w490 _]
                  tunnel: [w489 w576] -> w476
                  frame False {
                    n299 = local read "WhichPlayer"() -> (w486:i32)
                    n300 = Equal?(x=w490, y=0) -> (x = y?=w493:bool)
                    n301 = case shown="0, Default" w486 {
                      tunnel: [460139.0 1199628.0] -> w488
                      tunnel: [5866239.0 6678103.0] -> w487
                      frame 0, Default {
                        n302 = property on="P1's Score" class="DigNum (strict)"("NumText.BGColor"=u32 16711680 ("Label.Colors:BG Color")) -> ()  [unwired: 2 in, 2 out]
                        n303 = local read "P1's Score"() -> (w500:i32)
                        n304 = Subtract(x=w500, y=2) -> (x-y=w498:i32)
                        n305 = local write "P1's Score"(w498) -> ()
                      }
                      frame 1 {
                        n306 = property on="P2's Score" class="DigNum (strict)"("NumText.BGColor"=u32 16711680 ("Numeric Text.Text Colors:BG Color")) -> ()  [unwired: 2 in, 2 out]
                        n307 = local read "P2's Score"() -> (w506:i32)
                        n308 = Subtract(x=w506, y=2) -> (x-y=w504:i32)
                        n309 = local write "P2's Score"(w504) -> ()
                      }
                    }
                    n310 = case shown="True" w493 {
                      tunnel: w492 -> [w516 w547]
                      tunnel: w491 -> [w515 w546]
                      tunnel: w490 -> [w517 _]
                      tunnel: [T1."wait buttom" T1."ZeroSpread"] -> w489
                      tunnel: w488 -> [_ w540]
                      tunnel: w487 -> [w507 _]
                      tunnel: w486 -> [_ w539]
                      frame False {
                        n311 = flat-sequence {
                          tunnel: w517 -> [w520]
                          tunnel: w516 -> [w519]
                          tunnel: w515 -> [w518]
                          tunnel: [w520] -> w514
                          tunnel: [w519] -> w512
                          tunnel: [w518] -> w510
                          tunnel: w514 -> [w529]
                          tunnel: [w529] -> w513
                          tunnel: w512 -> [w528]
                          tunnel: [w528] -> w511
                          tunnel: w510 -> [w527]
                          tunnel: [w527] -> w509
                          tunnel: w513 -> [w536]
                          tunnel: w511 -> [w535]
                          tunnel: w509 -> [w534]
                          tunnel: w507 -> [w531]
                          frame #0 {
                            n312 = Number To Decimal String(number=w520) -> (decimal integer string=w523:string)  [unwired: 1 in]
                            n313 = local read "Show Map"() -> (w522:cluster{"Color Box":u32, "String":string}[][])
                            n314 = Bundle(16711680.0, w523) -> (w524:cluster{dbl, string})  [unwired: 1 in]
                            n315 = Replace Array Subset(array=w522, new element=w524, index (row)=w519, index (col)=w518) -> (w521:cluster{"Color Box":u32, "String":string}[][])
                            n316 = local write "Show Map"(w521) -> ()
                          }
                          frame #1 {
                            n317 = Wait Until Next ms Multiple(millisecond multiple=u32 1000) -> ()  [unwired: 1 out]
                          }
                          frame #2 {
                            w530 = u32 15132390 ("Label.Colors:BG Color")
                            n318 = local read "Show Map"() -> (w533:cluster{"Color Box":u32, "String":string}[][])
                            n319 = Number To Decimal String(number=w536) -> (decimal integer string=w537:string)  [unwired: 1 in]
                            n320 = Bundle(w531, w537) -> (w538:cluster{dbl, string})  [unwired: 1 in]
                            n321 = Replace Array Subset(array=w533, new element=w538, index (row)=w535, index (col)=w534) -> (w532:cluster{"Color Box":u32, "String":string}[][])
                            n322 = local write "Show Map"(w532) -> ()
                            n323 = property on="P1's Score" class="DigNum (strict)"("NumText.BGColor"=w530) -> ()  [unwired: 2 in, 2 out]
                            n324 = property on="P2's Score" class="DigNum (strict)"("NumText.BGColor"=w530) -> ()  [unwired: 2 in, 2 out]
                          }
                        }
                      }
                      frame True {
                        n325 = flat-sequence {
                          tunnel: w547 -> [w549]
                          tunnel: w546 -> [w548]
                          tunnel: [w549] -> w545
                          tunnel: [w548] -> w543
                          tunnel: w545 -> [w557]
                          tunnel: [w557] -> w544
                          tunnel: w543 -> [w556]
                          tunnel: [w556] -> w542
                          tunnel: w544 -> [w570]
                          tunnel: w542 -> [w569]
                          tunnel: w540 -> [w567]
                          tunnel: w539 -> [w559]
                          frame #0 {
                            n326 = local read "Show Map"() -> (w551:cluster{"Color Box":u32, "String":string}[][])
                            n327 = Bundle(16711680.0, "") -> (w552:cluster{dbl, string})  [unwired: 1 in]
                            n328 = Replace Array Subset(array=w551, new element=w552, index (row)=w549, index (col)=w548) -> (w550:cluster{"Color Box":u32, "String":string}[][])
                            n329 = local write "Show Map"(w550) -> ()
                          }
                          frame #1 {
                            n330 = Wait Until Next ms Multiple(millisecond multiple=u32 1000) -> ()  [unwired: 1 out]
                          }
                          frame #2 {
                            w558 = u32 15132390 ("Label.Colors:BG Color")
                            n331 = local read "Show Map"() -> (w571:cluster{"Color Box":u32, "String":string}[][])
                            n332 = Bundle(w567, "") -> (w572:cluster{dbl, string})  [unwired: 1 in]
                            n333 = Replace Array Subset(array=w571, new element=w572, index (row)=w570, index (col)=w569) -> (w568:cluster{"Color Box":u32, "String":string}[][])
                            n334 = local write "Show Map"(w568) -> ()
                            n335 = property on="P2's Score" class="DigNum (strict)"("NumText.BGColor"=w558) -> ()  [unwired: 2 in, 2 out]
                            n336 = property on="P1's Score" class="DigNum (strict)"("NumText.BGColor"=w558) -> ()  [unwired: 2 in, 2 out]
                            n337 = local read "Position"() -> (w566:i32[][])
                            n338 = local read "ZeroList"() -> (w561:i32[][])
                            n339 = Array Subset(array=w566, index (row)=w559, length (row)=1 ("length"), index (col)=0 ("index"), length (col)=2 ("length")) -> (w562:i32[][])
                            n340 = Build Array (concatenate)(w562, w561) -> (w560:i32[][])
                            n341 = local write "ZeroList"(w560) -> ()
                          }
                        }
                      }
                    }
                  }
                  frame True {
                    n342 = local read "WhichPlayer"() -> (w575:i32)
                    n343 = case shown="1" w575 {
                      tunnel: [5866239.0 6678103.0] -> w578
                      frame 0, Default {
                        n344 = local read "P1's Score"() -> (w591:i32)
                        n345 = Increment(x=w591) -> (x+1=w592:i32)
                        n346 = local write "P1's Score"(w592) -> ()
                      }
                      frame 1 {
                        n347 = local read "P2's Score"() -> (w594:i32)
                        n348 = Increment(x=w594) -> (x+1=w595:i32)
                        n349 = local write "P2's Score"(w595) -> ()
                      }
                    }
                    n350 = local read "Show Map"() -> (w580:cluster{"Color Box":u32, "String":string}[][])
                    n351 = Bundle(w578, "★") -> (w577:cluster{dbl, string})  [unwired: 1 in]
                    n352 = Replace Array Subset(array=w580, new element=w577, index (row)=w583, index (col)=w582) -> (w581:cluster{"Color Box":u32, "String":string}[][])
                    n353 = local write "Show Map"(w581) -> ()
                    n354 = flat-sequence {
                      tunnel: [w588] -> w574
                      frame #0 {
                        n355 = local read "Mines Remain"() -> (w586:i32)
                        n356 = Decrement(x=w586) -> (x-1=w587:i32)
                        n357 = local write "Mines Remain"(w587) -> ()
                      }
                      frame #1 {
                        n358 = local read "Mines Remain"() -> (w590:i32)
                        n359 = Equal?(x=w590, y=0) -> (x = y?=w588:bool)
                      }
                    }
                    n360 = case shown="False" w574 {
                      tunnel: [T1."wait buttom" T1."k"] -> w576
                      frame False {
                      }
                      frame True {
                      }
                    }
                  }
                }
              }
            }
          }
          frame "i" {
            n361 = flat-sequence {
              tunnel: [T1."ZeroSpread"] -> w597
              frame #0 {
                n362 = while {
                  stop <- "Start" stop-if-true
                }
                n363 = local write "Message"("Press START to play the game.") -> ()
              }
              frame #1 {
                n364 = Wait Until Next ms Multiple(millisecond multiple=u32 3000) -> ()  [unwired: 1 out]
                n365 = local write "Message"("Ready" ("Message")) -> ()
                n366 = property on="Start" class="Bool (strict)"("DisabledEnum"=T2."Disabled and Grayed Out" ("Disabled")) -> ()  [unwired: 2 in, 2 out]
              }
            }
          }
          frame "j" {
            n367 = for {
              N: 2 -> [_]
              i -> [w614]
              n368 = local read "Position"() -> (w617:i32[][])
              n369 = local read "BackMap"() -> (w612:i32[][])
              n370 = Index Array(array=w617, index (row) #1=w614, index (col) #1=0 ("index (row)"), index (row) #2=w614, index (col) #2=1 ("disabled index (col)")) -> (element #1=w611:i32, element #2=w610:i32)
              n371 = call "ZeroOrNot-V2.2.vi"("WhichPlayer"=w614, "index (col)"=w610, "index (row)"=w611, "BackMap"=w612) -> ("Numeric"=w613:dbl)  [unwired: 2 in]
              n372 = call "ToBackMap-V2.2.vi"("Column"=w610, "Row"=w611, "BackMap"=w612) -> ("String"=w609:string)  [unwired: 2 in, 1 out]
              n373 = local read "Show Map"() -> (w619:cluster{"Color Box":u32, "String":string}[][])
              n374 = Bundle("Numeric"=w613, "String"=w609) -> (w608:cluster{"Numeric":dbl, "String":string})  [unwired: 1 in]
              n375 = Replace Array Subset(array=w619, new element=w608, index (row)=w611, index (col)=w610) -> (w618:cluster{"Color Box":u32, "String":string}[][])
              n376 = local write "Show Map"(w618) -> ()
            }
            n377 = local write "NotFirstClick?"(TRUE ("NotFirstClick?")) -> ()
            n378 = local write "Message"("Go！\n\"Shift + #\" → reset map setting\n\"Shift + ! \" → reset all setting\n\"Shift + @\" → quit the game" ("Message")) -> ()
          }
          frame "k" {
            n379 = local read "P1's Score"() -> (w621:i32)
            n380 = local read "P2's Score"() -> (w620:i32)
            n381 = Equal?(x=w621, y=w620) -> (x = y?=w622:bool)
            n382 = case shown="False" w622 {
              tunnel: w621 -> [w626 _]
              tunnel: w620 -> [w625 _]
              frame False {
                n383 = Greater?(x=w626, y=w625) -> (0:w624:bool)
                n384 = case shown="False" w624 {
                  frame False {
                    n385 = local write "Message"("\"Shift + #\" → reset map setting\n\"Shift + ! \" → reset all setting\n\"Shift + @\" → quit the game") -> ()
                    n386 = One Button Dialog(message="All the mines are found.\nPlayer 2 wins！" ("Message")) -> ()  [unwired: 1 in, 1 out]
                  }
                  frame True {
                    n387 = local write "Message"("\"Shift + #\" → reset map setting\n\"Shift + ! \" → reset all setting\n\"Shift + @\" → quit the game") -> ()
                    n388 = One Button Dialog(message="All the mines are found.\nPlayer 1 wins！" ("Message")) -> ()  [unwired: 1 in, 1 out]
                  }
                }
              }
              frame True {
                n389 = local write "Message"("\"Shift + #\" → reset map setting\n\"Shift + ! \" → reset all setting\n\"Shift + @\" → quit the game") -> ()
                n390 = One Button Dialog(message="All the mines are found.\nTIE！" ("Message")) -> ()  [unwired: 1 in, 1 out]
              }
            }
          }
          frame "l" {
            n391 = local write "ButtonStringArray"(string[] []) -> ()
            n392 = local write "ButtonSetDone?"(FALSE ("ButtomSetDone?")) -> ()
            n393 = local write "ButtonArray"(i32[] [] ("ButtomArray")) -> ()
            n394 = local write "Buttom List"(string[][] [["", "P1", "P2"], ["↑", "", ""], ["←", "", ""], ["↓", "", ""], ["→", "", ""], ["☆", "", ""], ["★", "", ""]]) -> ()
            n395 = local write "Message"("【Set P1's key】 Press a key as ↑" ("Message")) -> ()
          }
          frame "u" {
          }
          frame "o" {
          }
          frame "spare" {
          }
          frame "ZeroSpread" {
            # "若Zerolist有新的點，則再進入此區找點，若沒有則去等待新的按鈕按下"
            # "將周圍0顆地雷的點旁邊的八個點打開"
            # "Zerolist放進原本Zerolist內周圍附近也沒有地雷的點"
            # "將Zerolist清空，之後要放入新發現周圍0顆地雷的點"
            # "點擊到周圍0顆地雷的點，就記錄進Zerolist，再先放到新的Array儲存"
            # "由於全域變數較晚才開始使用，因此需靠區域變數讀取"
            n396 = flat-sequence {
              tunnel: [w696] -> w644
              tunnel: [w693] -> w643
              tunnel: [w693] -> w642
              tunnel: [w704] -> w645
              tunnel: w644 -> [w705]
              tunnel: w643 -> [w714]
              tunnel: w642 -> [w710]
              frame #0 {
                n397 = local read "Show Map"() -> (w646:cluster{"Color Box":u32, "String":string}[][])
                n398 = local read "ZeroList"() -> (w648:i32[][])
                n399 = local write "ZeroListBefore"(w648) -> ()
                n400 = local read "BackMap"() -> (w647:i32[][])
                n401 = global write "BackMapGlobalV2.2.vi" "BackMap"(w647) -> ()
                n402 = global write "ShowMapGlobalV2.2.vi" "Show Map"(w646) -> ()
              }
              frame #1 {
                n403 = local write "ZeroList"(i32[][] []) -> ()
              }
              frame #2 {
                n404 = local read "ZeroListBefore"() -> (w650:i32[][])
                n405 = for {
                  tunnel: w650 -> [w652] mode=indexing
                  n406 = for {
                    N: 3 -> [_]
                    tunnel: w652 -> [w654]
                    i -> [w653]
                    n407 = for {
                      N: 3 -> [_]
                      tunnel: w654 -> [w669]
                      tunnel: w653 -> [w663]
                      i -> [w662]
                      n408 = local read "BackMap"() -> (w670:i32[][])
                      n409 = Index Array(array=w669, index #1=0 ("index"), index #2=1 ("index")) -> (element #1=w666:i32, element #2=w665:i32)
                      n410 = Decrement(x=w666) -> (x-1=w664:i32)
                      n411 = Decrement(x=w665) -> (x-1=w661:i32)
                      n412 = Add(x=w663, y=w664) -> (x+y=w657:i32)
                      n413 = Add(x=w661, y=w662) -> (x+y=w656:i32)
                      n414 = Index Array(array=w670, index (row)=w657, index (col)=w656) -> (element=w660:i32)
                      n415 = Equal?(x=-10, y=w660) -> (x = y?=w658:bool)
                      n416 = case shown="True" w658 {
                        tunnel: w657 -> [_ w674]
                        tunnel: w656 -> [_ w673]
                        frame False {
                        }
                        frame True {
                          n417 = local read "ZeroList"() -> (w675:i32[][])
                          n418 = Build Array(w674, w673) -> (w672:i32[])
                          n419 = Build Array (concatenate)(w675, w672) -> (w671:i32[][])
                          n420 = local write "ZeroList"(w671) -> ()
                        }
                      }
                    }
                  }
                }
              }
              frame #3 {
                n421 = local read "ZeroListBefore"() -> (w676:i32[][])
                n422 = for {
                  tunnel: w676 -> [w677] mode=indexing
                  n423 = for {
                    N: 3 -> [_]
                    tunnel: w677 -> [w680]
                    i -> [w679]
                    n424 = for {
                      N: 3 -> [_]
                      tunnel: w680 -> [w692]
                      tunnel: w679 -> [w686]
                      i -> [w685]
                      n425 = Index Array(array=w692, index #1=0 ("index"), index #2=1 ("index")) -> (element #1=w689:i32, element #2=w688:i32)
                      n426 = Decrement(x=w689) -> (x-1=w687:i32)
                      n427 = Decrement(x=w688) -> (x-1=w684:i32)
                      n428 = Add(x=w686, y=w687) -> (x+y=w683:i32)
                      n429 = Add(x=w684, y=w685) -> (x+y=w682:i32)
                      n430 = call "Uncover-V2.2.vi"("index (col)"=w682, "index (row)"=w683) -> ()  [unwired: 3 in]
                    }
                  }
                }
              }
              frame #4 {
                n431 = global read "BackMapGlobalV2.2.vi" "BackMap"() -> (w695:i32[][])
                n432 = local write "BackMap"(w695) -> ()
                n433 = global read "ShowMapGlobalV2.2.vi" "Show Map"() -> (w694:cluster{"Color Box":u32, "String":string}[][])
                n434 = local write "Show Map"(w694) -> ()
                n435 = local read "ZeroList"() -> (w703:i32[][])
                n436 = Array Size(array=w703) -> (size(s)=w702:i32[])
                n437 = Index Array(array=w702, index=0) -> (element=w700:i32)
                n438 = Equal?(x=w700, y=0) -> (x = y?=w693:bool)
                n439 = Select(t=T1."wait buttom", s=w693, f=T1."ZeroSpread") -> (s? t:f=w696:T1)
              }
              frame #5 {
                n440 = local read "NotFirstClick?"() -> (w712:bool)
                n441 = And(x=w714, y=w712) -> (x .and. y?=w713:bool)
                n442 = Equal?(x=w710, y=TRUE) -> (x = y?=w706:bool)
                n443 = case shown="True" w713 {
                  frame False {
                  }
                  frame True {
                    n444 = local read "BackMap"() -> (w722:i32[][])
                    n445 = local read "Show Map"() -> (w721:cluster{"Color Box":u32, "String":string}[][])
                    n446 = local read "WhichPlayer"() -> (w726:i32)
                    n447 = local read "Position"() -> (w727:i32[][])
                    n448 = call "AfterZeroSpreadColor-V2.2.vi"("BackMap"=w722, "WhichPlayer"=w726, "Position"=w727) -> ("col"=w719:i32, "row"=w720:i32, "Numeric"=w723:dbl)  [unwired: 1 in]
                    n449 = Index Array(array=w721, index (row)=w720, index (col)=w719) -> (element=w725:cluster{"Color Box":u32, "String":string})
                    n450 = Unbundle(w725) -> ("String"=w724:string)  [unwired: 1 out]
                    n451 = Bundle("Numeric"=w723, "String"=w724) -> (w718:cluster{"Numeric":dbl, "String":string})  [unwired: 1 in]
                    n452 = Replace Array Subset(array=w721, new element=w718, index (row)=w720, index (col)=w719) -> (w717:cluster{"Color Box":u32, "String":string}[][])
                    n453 = local write "Show Map"(w717) -> ()
                  }
                }
                n454 = Equal?(x=w712, y=FALSE) -> (x = y?=w707:bool)
                n455 = And(x=w707, y=w706) -> (x .and. y?=w708:bool)
                n456 = case shown="True" w708 {
                  tunnel: w705 -> [w715 _]
                  tunnel: [w715 T1."j"] -> w704
                  frame False {
                  }
                  frame True {
                  }
                }
              }
            }
          }
        }
      }
    }
  }
